vi "Write DeviceTerm.vi"(8 "error in (no error)":errorcluster, 10 "deviceTerm":string, 11 "CCD in":refnum<class "CCD.lvclass">) -> (0 "error out":errorcluster, 3 "CCD out":refnum<class "CCD.lvclass">)   [LabVIEW 2023, in "CCD.lvclass"]
doc: "Sets the device term after init."
uses:
  CCD.lvclass
  GenericDevice/GenericDevice.lvclass
panel:
  # "Connector Pane"
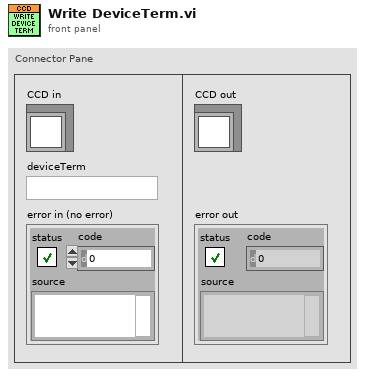
[diagram p1: front panel]
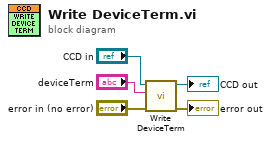
[diagram p0: block diagram]
diagram:
  n1 = call-parent "Write DeviceTerm.vi"("error in (no error)"="error in (no error)", "deviceTerm"="deviceTerm", "GenericDevice in"="CCD in") -> ("error out"=→"error out":errorcluster, "GenericDevice out"=→"CCD out":refnum<class "CCD.lvclass">)  [unwired: 7 in]
